vi "EEI EXP4b.vi"() -> ()   [LabVIEW 2020]
panel:
  out "Factorial using while loop":i32
  in  "Numeric3":i32
  out "Factorial using for loop":i32
  in  "N value":i32
  out "current time":timestamp
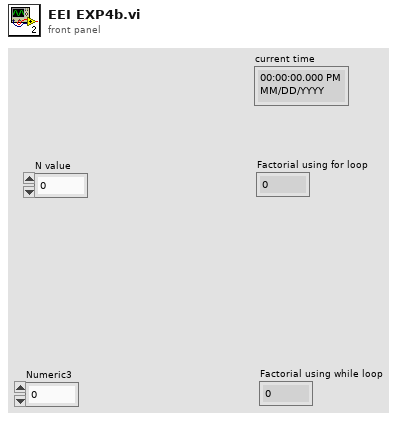
[diagram p1: front panel]
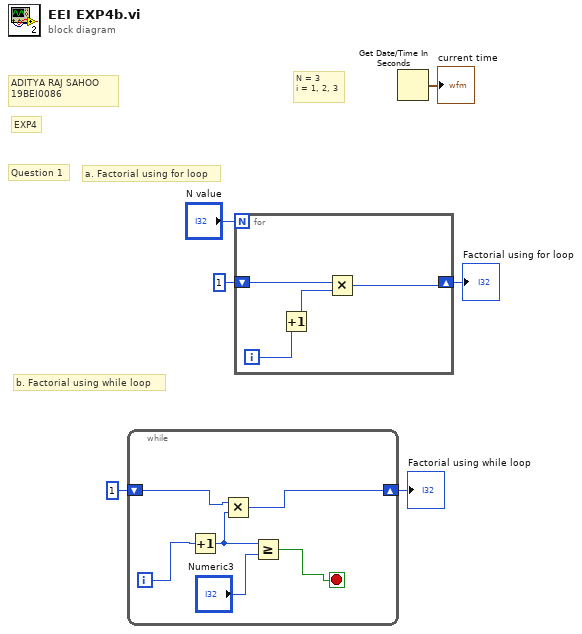
[diagram p0: block diagram]
diagram:
  # "b. Factorial using while loop"
  # "EXP4"
  # "a. Factorial using for loop"
  # "ADITYA RAJ SAHOO\n19BEI0086"
  # "Question 1"
  # "N = 3\ni = 1, 2, 3"
  n1 = while {
    shift-right: [w11] -> w1
    shift-left: 1 -> [w12]
    i -> [w10]
    stop <- w9 stop-if-true
    n2 = Increment(x=w10) -> (x+1=w8:i32)
    n3 = Multiply(x=w12, y=w8) -> (x*y=w11:i32)
    n4 = Greater Or Equal?(x=w8, y="Numeric3") -> (x >= y?=w9:bool)
  }
  "Factorial using while loop" <- w1
  n5 = for {
    N: "N value" -> [_]
    shift-right: [w13] -> w3
    shift-left: 1 -> [w14]
    i -> [w16]
    n6 = Increment(x=w16) -> (x+1=w15:i32)
    n7 = Multiply(x=w14, y=w15) -> (x*y=w13:i32)
  }
  "Factorial using for loop" <- w3
  n8 = Get Date/Time In Seconds() -> (seconds since 1Jan1904=→"current time":timestamp)
